vi "CRC16.vi"(11 "Array":u8[](array[numeric])) -> (3 "Numeric":u16)   [LabVIEW 2021]
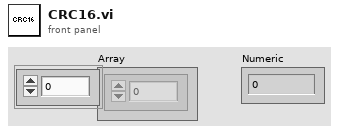
[diagram p1: front panel]
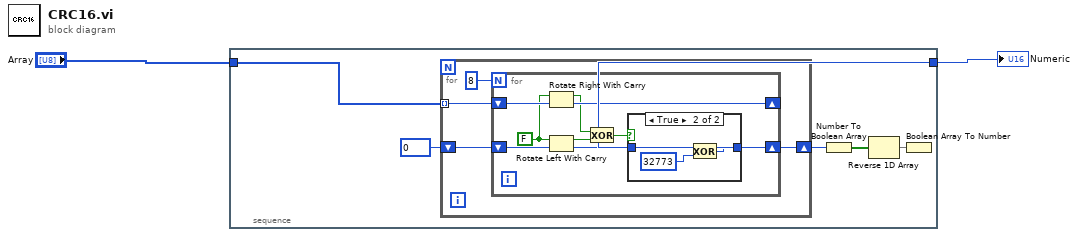
[diagram p0: block diagram]
diagram:
  n1 = stacked-sequence {
    tunnel: [w3] -> w2
    tunnel: "Array" -> [w4]
    frame #0 {
      n2 = for {
        shift-right: [w9] -> w8
        shift-left: u16 0 ("Initial CRC") -> [w11]
        tunnel: w4 -> [w10] mode=indexing
        n3 = for {
          N: 8 -> [_]
          shift-right: [w17] -> w9
          shift-left: w11 -> [w14]
          shift-right: [w20] -> _
          shift-left: w10 -> [w21]
          w15 = FALSE ("carry")
          n4 = Rotate Right With Carry(2:w21, 3:w15) -> (0:w20:u8, 1:w19:bool)
          n5 = Rotate Left With Carry(2:w14, 3:w15) -> (0:w13:u16, 1:w16:bool)
          n6 = Exclusive Or(1:w16, 2:w19) -> (0:w18:bool)
          n7 = case shown="True" w18 {
            tunnel: w13 -> [w22 w25]
            tunnel: [w22 w24] -> w17
            frame False {
            }
            frame True {
              n8 = Exclusive Or(1:u16 32773 ("Polynomial"), 2:w25) -> (0:w24:u16)
            }
          }
        }
      }
      n9 = Number To Boolean Array(number=w8) -> (Boolean array=w7:bool[])
      n10 = Reverse 1D Array(array=w7) -> (reversed array=w6:bool[])
      n11 = Boolean Array To Number(Boolean array=w6) -> (number=w3:u16)
    }
  }
  "Numeric" <- w2
